vi "beep by freq.vi"(8 "error in (no error)":errorcluster, 9 "use system alert? (T)":bool, 10 "duration (msec)":u32=350, 11 "frequency (Hz)":u32=700) -> (0 "error out":errorcluster)   [LabVIEW 2013]
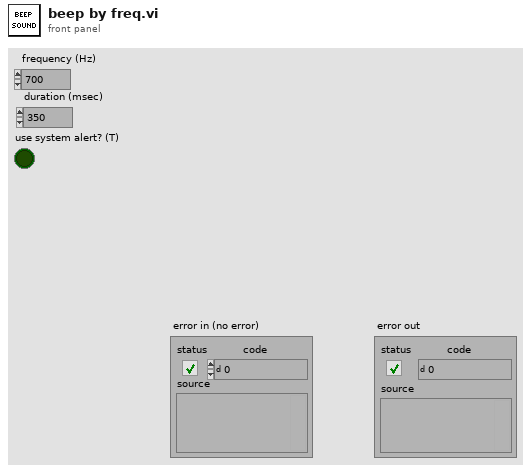
[diagram p1: front panel]
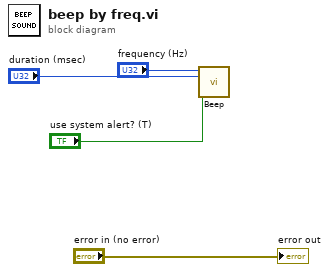
[diagram p0: block diagram]
diagram:
  n1 = call <vilib>:"Beep.vi"("use system alert? (T)"="use system alert? (T)", "duration (msec)"="duration (msec)", "frequency (Hz)"="frequency (Hz)") -> ()  [unwired: 9 in]
  "error out" <- "error in (no error)"
